vi "multi emitter_Personality_5785_FPGA_2_x_1_6G.vi"() -> ()   [LabVIEW 2021]
uses:
  <instrlib>/_niInstr/Streaming/v1/Common/Stream State.ctl
  <vilib>/Platform/TimedLoop/XDataNode/timing_clust.ctl
  <vilib>/Platform/TimedLoop/XDataNode/nitl_modes.ctl
  <vilib>/Platform/TimedLoop/XDataNode/wakeup.ctl
  <instrlib>/FlexRIO/API/FPGA/v1/Types/Start Trigger IO Resources.ctl
  <vilib>/rvi/Emulation/niFpgaSctlEmulationGetInTimedLoop.vi
  <vilib>/rvi/Emulation/niFpgaEmulationReportErrorSimple.vi
  <vilib>/rvi/Emulation/niFpgaGetClockAttributes.vi
  <vilib>/rvi/Emulation/niFpgaCriticalErrorInLSC.vi
  7192f61d-e408-4cca-baff-cb10c33219c0.vi
  <vilib>/rvi/interface/RandomDataEmulation/nirviRandomDataMultiElementFPGAFIFO.vi
  <instcachedir>/0/nirviRandomDataMultiElementFPGAFIFO_3E9965BA1FAD4E7B8DABA31768A09B1F.lvgen/nirviRandomDataMultiElementFPGAFIFO_3E9965BA1FAD4E7B8DABA31768A09B1F_000.vi
  <vilib>/rvi/interface/RandomDataEmulation/niFpgaRandomDataHandleErrors.vi
  <instrlib>/_niInstr/DSP/v1/FPGA/Public/Sub VIs/HB Interpolator/Halfband Interpolator - IQ - 8 SPC - 2x OC.vi
  <vilib>/rvi/eio/common/nirviEmuTemplateMethod_errors.vi
  <vilib>/Platform/TimedLoop/XDataNode/XDataNode.xnode
  <vilib>/rvi/DataTransferAndStorage/Container/XNode/niFpgaContainer.xnode
  <vilib>/rvi/interface/RandomDataEmulation/nirviRandomDataFpgaMultiElementTemplate.vi
  <vilib>/eio/EIONode/EIONode.xnode
  <vilib>/Platform/TimedLoop/XDataNode/XDNodeRunTimeDep.lvlib
  <instrlib>/_niInstr/Streaming/v1/FPGA/niInstr Streaming v1 FPGA.lvlib
  <instrlib>/FlexRIO/API/FPGA/v1/FlexRIO API FPGA v1.lvlib
  <instrlib>/FlexRIO/API/FPGA/v1/IO/NI5785/FlexRIO 5785 FPGA v1.lvlib
  <instrlib>/_niInstr/DSP/v1/FPGA/niInstr DSP v1 FPGA.lvlib
  <instrlib>/_niInstr/Basic Elements/v1/FPGA/niInstr Basic Elements v1 FPGA.lvlib
  <instrlib>/_niInstr/Streaming/v1/Common/niInstr Streaming v1 Common.lvlib
panel:
  out "pulse TX status 2":T1
  out "pulse TX status":T1
  in  "reset system clock":bool
  in  "User-defined Start Trigger - AO":bool
  in  "flexrio.trigger.start.cfg 1":u16
  out "written elements":u64
  out "IO Socket\\AO Ready For Input":bool
  in  "stream.request state 1":T2
  in  "stream.num samples 1":u64
  out "stream.metadata 1":u64
  out "stream.samples transferred 1":u64
  out "stream.state 1":T2
  out "flexrio.module.io ready 0":bool
  out "flexrio.module.io error 0":i32
  out "flexrio.module.data valid 0":bool
  # "Data Path Configuration"
  # "AI Trigger Configuration"
  # "AI Stream Configuration"
  # "AO Stream Configuration"
  # "Module Status"
  # "AO Buffer Configuration"
  # "Device Utilization\n---------------------------\nTotal Slices: 62.6% (18977 out of 30300)\nSlice Registers: 23.8% (115206 out of 484800)\nSlice LUTs: 38.2% (92532 out of 242400)\nBlock RAMs: 56.8% (341 out of 600)\nDSP48s: 0.3% (6 out of 1920)\n\nNote: Utilization numbers are for the KU040. Exact values will vary for the KU060 and KU035."
  # "User-defined Controls"
  # "AO Trigger Configuration"
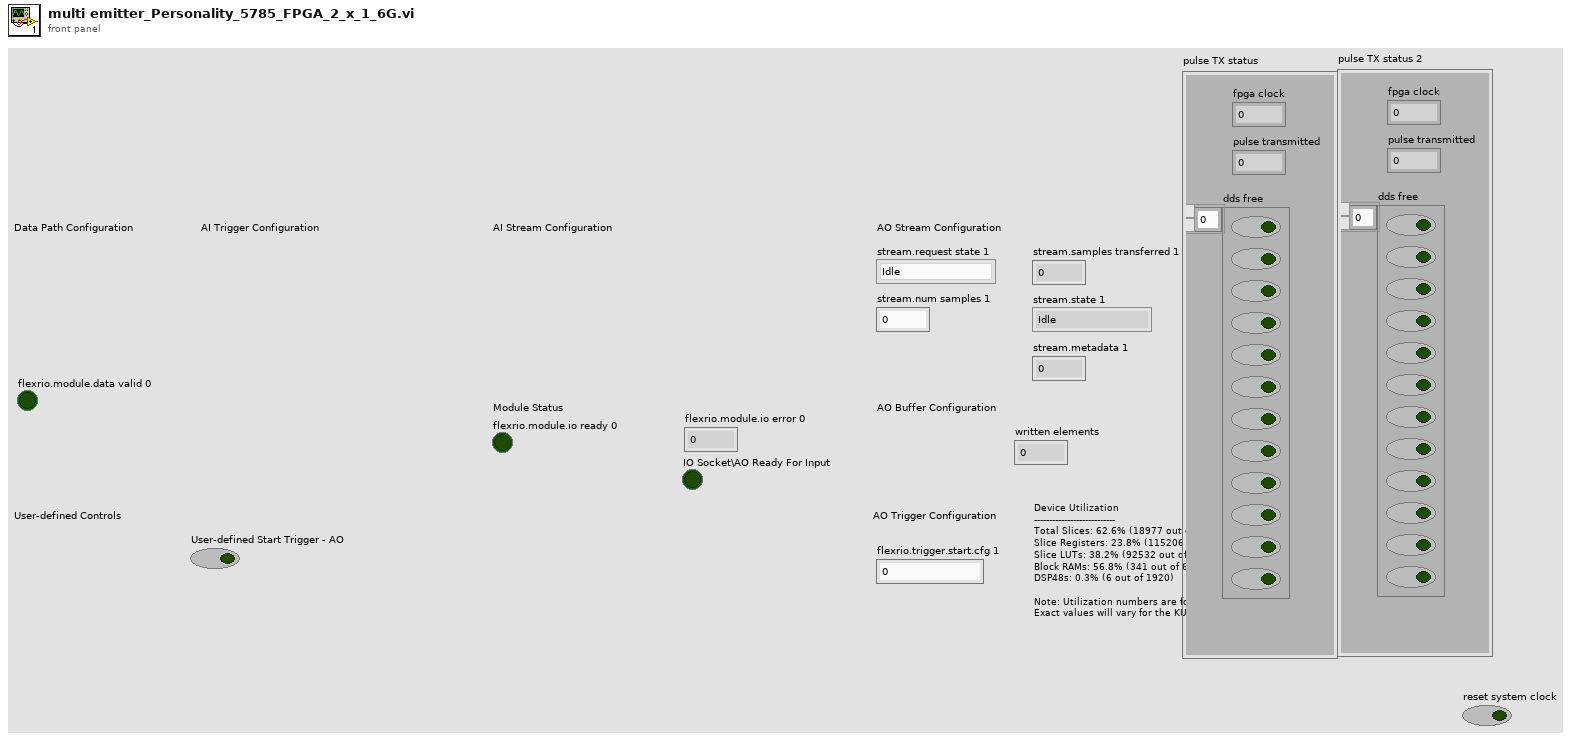
[diagram p1: front panel]
types:
  T1 = cluster{"fpga clock":u64, "pulse transmitted":u32, "dds free":bool[]}
  T2 = typedef "niInstr Streaming v1 Common.lvlib/Stream State.ctl" = enum8{"Idle", "Finite Transfer", "Continuous", "Done", "Error", "Not Ready", "Cancel"}
  T3 = typedef "XDNodeRunTimeDep.lvlib/timing_clust.ctl" = cluster{"Expected End [f-1]":u64, "Actual End [f-1]":u64, "Finished Late? [f-1]":bool, "Expected End [i-1]":u64, "Actual End [i-1]":u64, "Finished Late? [i-1]":bool, "Expected Start [i]":u64, "Actual Start [i]":u64, "Expected Start [f]":u64, "Actual Start [f]":u64, "Source Name":string, "Structure Name":string, "Period":i64, "Deadline":i64, "Offset":i64, "Start":i64, "Priority":i32, "Timeout":i32, "Mode":T4, "Wakeup Reason":T5, "Error":errorcluster, "Source Type":string, "Secondary Source Type":string, "Global End Time":u64, "Global Start Time":u64, "Frame Duration":u64, "Iteration Duration":u64, "Assigned CPU":i32, "I/O Scan Engine Mode":u32}
  T4 = typedef "XDNodeRunTimeDep.lvlib/nitl_modes.ctl" = enum32{"No Change", "Process missed periods, maintain original phase", "Discard missed periods, maintain original phase", "Process missed periods, ignore original phase", "Discard missed periods, ignore original phase"}
  T5 = typedef "XDNodeRunTimeDep.lvlib/wakeup.ctl" = enum32{"Normal", "Aborted", "Asynchronous wakeup", "Timing source error", "Timed loop error", "Timeout"}
  T6 = typedef "FlexRIO API FPGA v1.lvlib/Start Trigger IO Resources.ctl" = cluster{"start trigger":refnum<k21>, "started event":refnum<k21>, "start trigger for export":refnum<k21>, "start trigger for tclk":refnum<k21>}
  T7 = typedef "FlexRIO API FPGA v1.lvlib/Start Trigger Control.ctl" = cluster{"arm start":bool, "done":bool}
  T8 = typedef "niInstr DSP v1 Shared.lvlib/IQ Data.ctl" = cluster{"I":fxp<+/-,18,1>, "Q":fxp<+/-,18,1>, "overflow":bool}
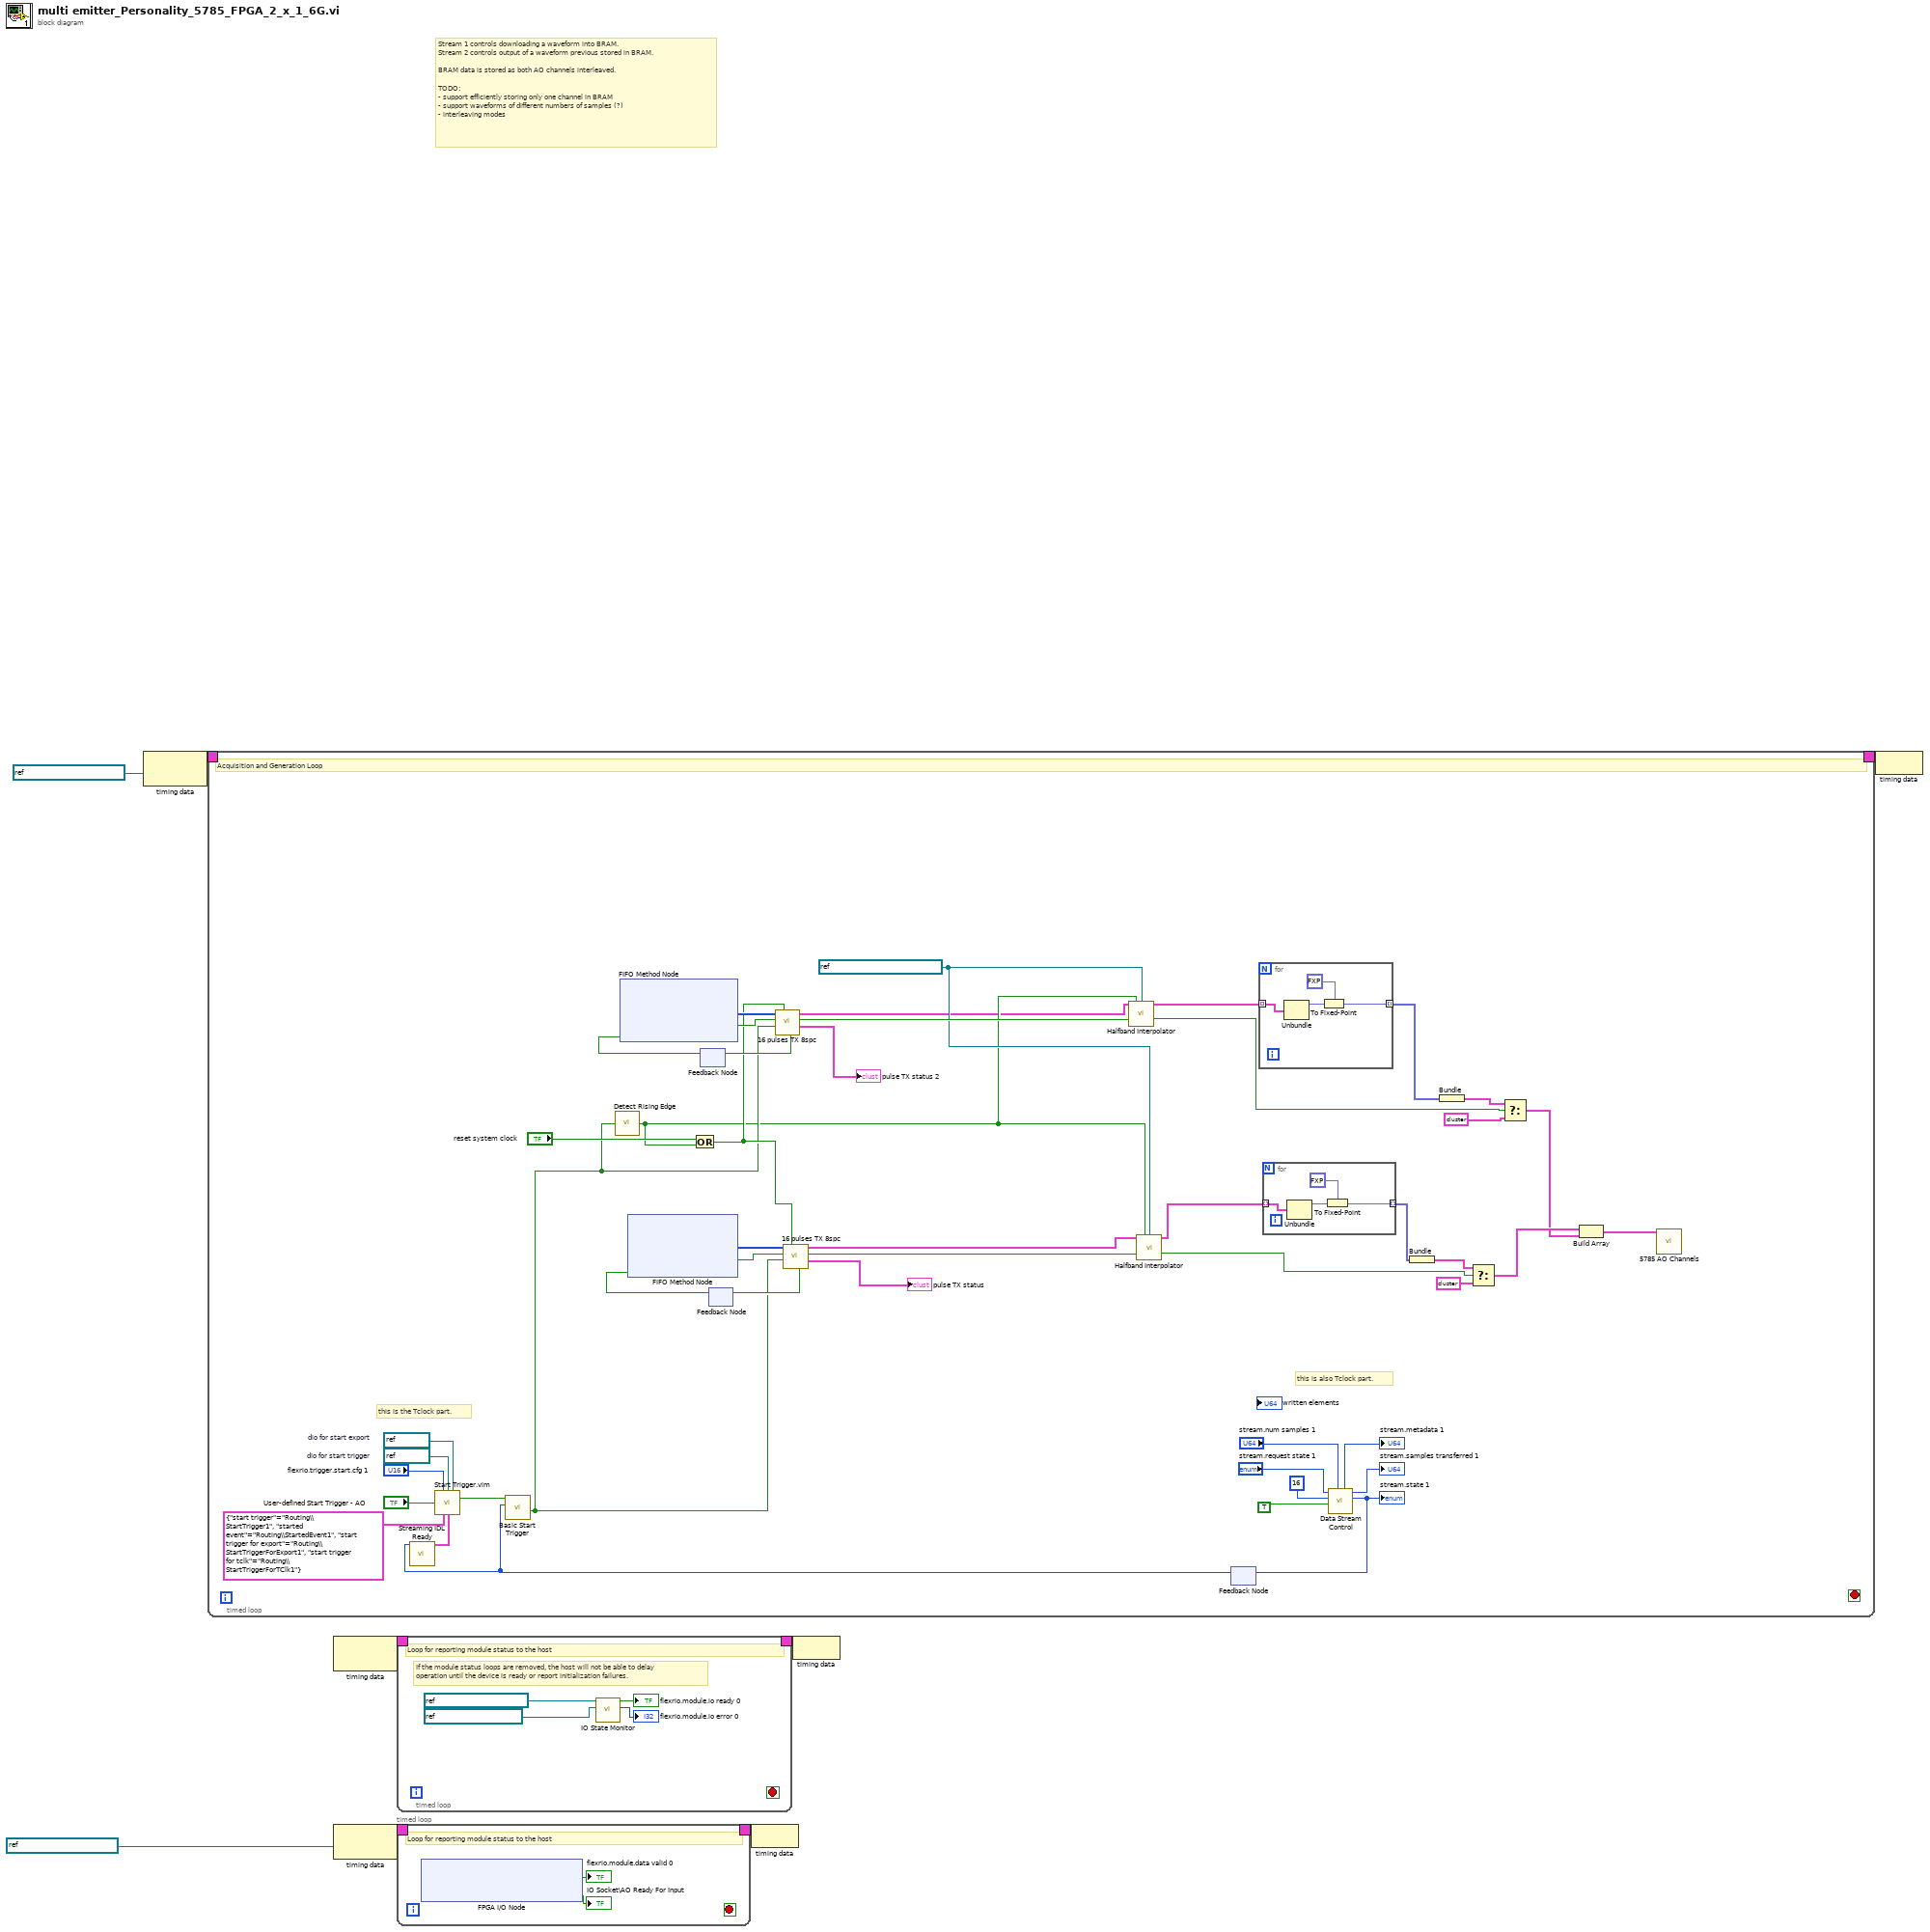
[diagram p0: block diagram]
diagram:
  # "Stream 1 controls downloading a waveform into BRAM.\nStream 2 controls output of a waveform previous stored in BRAM.\n\nBRAM data is stored as both AO channels interleaved.\n\nTODO:\n- support efficiently storing only one channel in BRAM\n- support waveforms of different numbers of samples (?)\n- interleaving modes"
  n1 = node-c288(refnum<k21> "IO Socket\\Data Clock" ("Source Name")) -> (w8:T3)
  n2 = timed-loop {
    timing: w8 -> [_]
    timing-out: [_] -> w7
    stop <- _ stop-if-true
    w27 = refnum<k21> "IO Socket\\Data Clock 2x" ("Source Name")
    w44 = refnum<k21> "DIO 2"  # dio for start trigger
    w43 = refnum<k21> "DIO 3"  # dio for start export
    # "this is also Tclock part."
    # "this is the Tclock part."
    # "Acquisition and Generation Loop"
    n3 = feedback #1() -> (w32:bool)  [unwired: 1 in]
    n4 = xnode ("FIFO Method Node")("Ready for Output"=w32) -> ("Element"=w34:u64[], "Output Valid"=w30:bool)  [unwired: 1 in, 1 out]
    n5 = feedback #2() -> (w36:bool)  [unwired: 1 in]
    n6 = xnode ("FIFO Method Node")("Ready for Output"=w36) -> ("Element"=w35:u64[], "Output Valid"=w23:bool)  [unwired: 1 in, 1 out]
    n7 = feedback #3() -> (w41:T2)  [unwired: 1 in]
    n8 = call <instrlib>:"Streaming IDL Ready.vi"("stream.state"=w41) -> ("start trigger control"=w46:T7)  [unwired: 10 in]
    n9 = call "Start Trigger.vim"("flexrio.trigger.start.cfg 0"="flexrio.trigger.start.cfg 1", "dio start"=w44, "dio for start export"=w43, "user-defined start trigger"="User-defined Start Trigger - AO", "trigger io resources"=T6 {"start trigger"="Routing\\StartTrigger1", "started event"="Routing\\StartedEvent1", "start trigger for export"="Routing\\StartTriggerForExport1", "start trigger for tclk"="Routing\\StartTriggerForTClk1"}, "start trigger control"=w46) -> ("conditioned start trigger"=w45:bool)  [unwired: 7 in, 2 out]
    n10 = call <instrlib>:"Basic Start Trigger.vi"("stream.state"=w41, "start trigger"=w45) -> ("data valid"=w24:bool)  [unwired: 9 in]
    n11 = call <instrlib>:"Detect Rising Edge.vi"("signal"=w24) -> ("edge detected"=w13:bool)  [unwired: 14 in]
    n12 = Or(x="reset system clock", y=w13) -> (x .or. y?=w25:bool)
    n13 = call "16 pulses TX 8spc.vi"("reset system clock"=w25, "IQ_run"=w24, "PDW input Valid"=w30, "array PDW"=w34) -> ("pulse TX status"=→"pulse TX status 2":T1, "output valid"=w33:bool, "IQ out"=w10:T8[], "ready for input"=w31:bool)  [unwired: 4 in]
    n14 = feedback-in #1(w31) -> ()
    n15 = call "16 pulses TX 8spc.vi"("reset system clock"=w25, "IQ_run"=w24, "PDW input Valid"=w23, "array PDW"=w35) -> ("pulse TX status"=→"pulse TX status":T1, "output valid"=w20:bool, "IQ out"=w12:T8[], "ready for input"=w37:bool)  [unwired: 4 in]
    n16 = feedback-in #2(w37) -> ()
    n17 = call-poly <instrlib>:"Halfband Interpolator.vi"("data in"=w10, "reset"=w13, "clock x 2"=w27, "input valid"=w33) -> ("data out"=w28:T8[], "output valid"=w29:bool)  [unwired: 8 in, 2 out]
    n18 = call-poly <instrlib>:"Halfband Interpolator.vi"("data in"=w12, "reset"=w13, "clock x 2"=w27, "input valid"=w20) -> ("data out"=w39:T8[], "output valid"=w38:bool)  [unwired: 8 in, 2 out]
    n19 = for {
      tunnel: w28 -> [w59] mode=indexing
      tunnel: [w56] -> w21 mode=indexing
      n20 = Unbundle(w59) -> ("I"=w58:fxp<+/-,18,1>)  [unwired: 2 out]
      n21 = To Fixed-Point(fixed-point type=fxp<+/-,12,1> 0.0 ("element"), number=w58) -> (fixed-point=w56:fxp<+/-,12,1>)
    }
    n22 = for {
      tunnel: w39 -> [w63] mode=indexing
      tunnel: [w60] -> w22 mode=indexing
      n23 = Unbundle(w63) -> ("I"=w62:fxp<+/-,18,1>)  [unwired: 2 out]
      n24 = To Fixed-Point(fixed-point type=fxp<+/-,12,1> 0.0 ("element"), number=w62) -> (fixed-point=w60:fxp<+/-,12,1>)
    }
    n25 = call <instrlib>:"Data Stream Control.vi"("stream.num samples 0"="stream.num samples 1", "data valid"=TRUE, "element count"=u16 16, "stream.request state 0"="stream.request state 1") -> ("stream.state 0"=w48:T2, "stream.samples transferred 0"=→"stream.samples transferred 1":u64, "stream.metadata 0"=→"stream.metadata 1":u64)  [unwired: 3 in, 2 out]
    "stream.state 1" <- w48
    n26 = feedback-in #3(w48) -> ()
    n27 = Bundle(w22) -> (w19:cluster{fxp<+/-,12,1>[]})  [unwired: 1 in]
    n28 = Bundle(w21) -> (w15:cluster{fxp<+/-,12,1>[]})  [unwired: 1 in]
    n29 = Select(t=w19, s=w38, f=cluster{fxp<+/-,12,1>[]} {[0.0, 0.0, 0.0, 0.0, 0.0, 0.0, 0.0, 0.0, 0.0, 0.0, 0.0, 0.0, 0.0, 0.0, 0.0, 0.0]}) -> (s? t:f=w18:cluster{fxp<+/-,12,1>[]})
    n30 = Select(t=w15, s=w29, f=cluster{fxp<+/-,12,1>[]} {[0.0, 0.0, 0.0, 0.0, 0.0, 0.0, 0.0, 0.0, 0.0, 0.0, 0.0, 0.0, 0.0, 0.0, 0.0, 0.0]}) -> (s? t:f=w14:cluster{fxp<+/-,12,1>[]})
    n31 = Build Array(w18, w14) -> (w53:cluster{fxp<+/-,12,1>[]}[])
    n32 = call <instrlib>:"5785 AO Channels.vi"("all channels"=w53) -> ()  [unwired: 15 in]
  }
  n33 = node-c288() -> (w5:T3)  [unwired: 1 in]
  n34 = node-c288(refnum<k21> "IO Socket\\Data Clock" ("Source Name")) -> (w3:T3)
  n35 = timed-loop {
    timing: w5 -> [_]
    timing-out: [_] -> w4
    stop <- _ stop-if-true
    # "If the module status loops are removed, the host will not be able to delay operation until the device is ready or report initialization failures."
    # "Loop for reporting module status to the host"
    n36 = call <instrlib>:"IO State Monitor.vi"("io error resource"=refnum<k21> "IO Socket\\IO Error" ("FPGA I/O In"), "io ready resource"=refnum<k21> "IO Socket\\IO Ready" ("FPGA I/O In")) -> ("flexrio.module.io error 0"=→"flexrio.module.io error 0":i32, "flexrio.module.io ready 0"=→"flexrio.module.io ready 0":bool)  [unwired: 8 in]
  }
  n37 = timed-loop {
    timing: w3 -> [_]
    timing-out: [_] -> w2
    stop <- _ stop-if-true
    # "Loop for reporting module status to the host"
    n38 = xnode "FPGA I/O Node"() -> ("IO Socket\\AI Data Valid"=→"flexrio.module.data valid 0":bool, "IO Socket\\AO Ready For Input"=→"IO Socket\\AO Ready For Input":bool)  [unwired: 2 in, 2 out]
  }
  n39 = node-c288(w2) -> ()
  n40 = node-c288(w4) -> ()
  n41 = node-c288(w7) -> ()
